vi "subVI_Create Relative Timestamp.vi"(8 "error in (no error)":errorcluster, 11 "waveform in":waveform(dbl)) -> (0 "error out":errorcluster, 3 "waveform out":waveform(dbl))   [LabVIEW 2010]
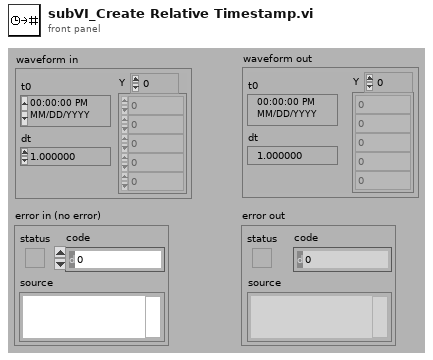
[diagram p1: front panel]
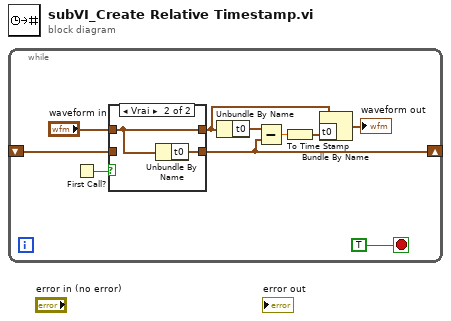
[diagram p0: block diagram]
diagram:
  n1 = while {
    shift-right: [w5] -> _
    shift-left: _ -> [w4]
    stop <- TRUE stop-if-true
    n2 = First Call?() -> (First Call?: T/F=w6:bool)
    n3 = case shown="Vrai" w6 {
      tunnel: "waveform in" -> [w11 w13]
      tunnel: [w12 w14] -> w5
      tunnel: w4 -> [w12 _]
      tunnel: [w11 w13] -> w1
      frame False {
      }
      frame True {
        n4 = Unbundle By Name(w13) -> ("t0"=w14:timestamp)
      }
    }
    n5 = Unbundle By Name(w1) -> ("t0"=w7:timestamp)
    n6 = Subtract(x=w7, y=w5) -> (x-y=w9:dbl)
    n7 = To Time Stamp(1:w9) -> (0:w10:timestamp)
    n8 = Bundle By Name(cluster=w1, "t0"=w10) -> (→"waveform out":waveform(dbl))
  }
